vi "串口通信.vi"() -> ()   [LabVIEW 2014]
uses:
  <vilib>/Instr/_visa.llb/VISA Configure Serial Port (Instr).vi
  <vilib>/Utility/file.llb/Write To Spreadsheet File (string).vi
  <vilib>/sound2/lvsound2.llb/Sound File Read Open.vi
  <vilib>/sound2/lvsound2.llb/Sound File Read (DBL).vi
panel:
  in  "写入缓冲区":string="！0000?"
  in  "选项卡控件":enum32{"曲线图", "记录表", "设置"}(tab)
  out "湿度曲线 1":dbl(graph)
  out "温度曲线 1":dbl(graph)
  out "湿度曲线 2":dbl(graph)
  out "温度曲线 3":dbl(graph)
  out "湿度曲线 3":dbl(graph)
  out "温度曲线 2":dbl(graph)
  out "警报":bool
  out "湿度计 3":dbl(knob) scale=0.0..100.0
  out "警报":bool
  out "表格":string[][](table)
  out "湿度计  1":dbl(knob) scale=0.0..100.0
  out "湿度计 2":dbl(knob) scale=0.0..100.0
  out "温度计 1":dbl(slide) scale=0.0..100.0
  out "温度计 2":dbl(slide) scale=0.0..100.0
  out "温度计 3":dbl(slide) scale=0.0..100.0
  in  "创建表格":bool
  in  "选项卡控件 2":enum32{"开关选项", "上下限设置", "设置", "开发人员选项"}(tab)
  in  "自动模式":bool=TRUE
  in  "加热棒":bool
  in  "制冷片":bool
  in  "风扇":bool
  in  "报警灯":bool
  in  "湿度下限":u8(slide) scale=0.0..100.0
  in  "温度上限":u8(slide)=100 scale=0.0..100.0
  in  "温度下限":u8(slide) scale=0.0..100.0
  in  "湿度上限":u8(slide)=100 scale=0.0..100.0
  in  "Recipients 2":string="971661949@qq.com" caption="报警邮箱"
  in  "打开串口":bool
  in  "file path (dialog if empty)":path=path "d:/data.xls" caption="报表路径"
  in  "VISA resource name":refnum<visa-resource-name> caption="选择串口"
  in  "停止":bool
  out "火焰状态":string
  out "数据 4":string
  out "烟雾状态":string
  out "连接的字符串":string
  out "外人检测":string
  out "进入检测":string
  out "警报":bool
  in  "温湿度报警":bool
  in  "提示开关":bool=TRUE
  out "当前时间":timestamp format="%<%H:%M\n%Y年%m月%d>T日"
  out "数据 3":string
  out "输出数组":string[][](array[string])
  out "温度数据3":string
  out "湿度数据3":string
  out "数值 2":u8
  out "数据传输":i32
  out "湿度数据2":string
  out "温度数据2":string
  out "数据 2":string
  out "湿度数据1":string
  out "温度数据1":string
  out "数据 1":string
  in  "baud rate (9600)":u32=9600 caption="波特率(9600)"
  in  "parity (0:none)":enum16{"None", "Odd", "Even", "Mark", "Space"}(ring) caption="奇偶（0:无）"
  in  "data bits (8)":u16=8 caption="数据比特(8)" min=5 max=8 step=1
  in  "stop bits (10: 1 bit)":u16(ring)=10 caption="停止位（10: 1位）" items=["1.0"=10, "1.5"=15, "2.0"=20]
  in  "flow control (0:none)":u16(ring) caption="流控制（0:无）" items=["无", "XON/XOFF", "RTS/CTS", "XON/XOFF & RTS/CTS", "DTR/DSR", "XON/XOFF & DTR/DSR"]
  # "库房监控"
  # "使用图表实时反馈\n温湿度状况"
  # "这里有很全面的数据\n还可以将数据以表格形式保存到电脑"
  # "请在设置中选择串口位置"
  # "不要忘记核对信息哦"
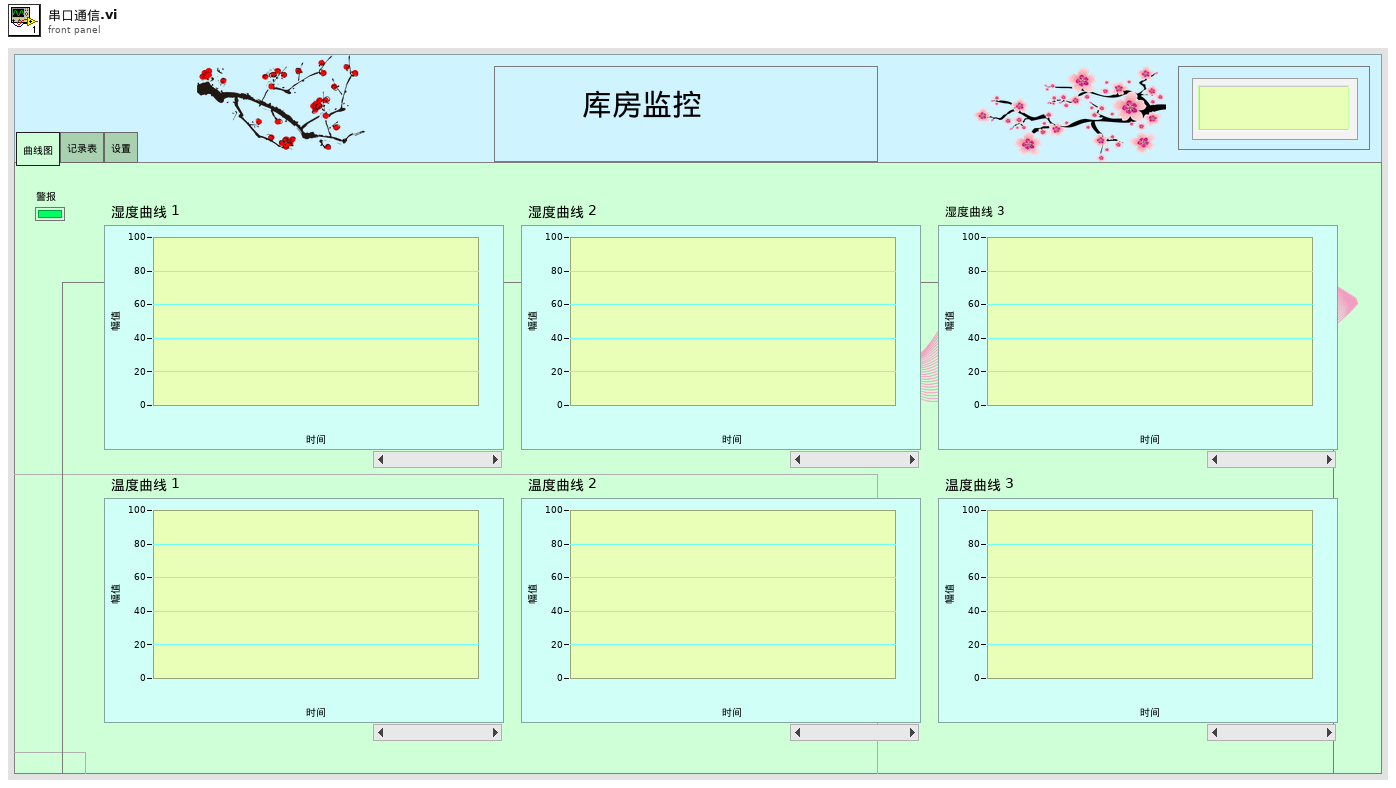
[diagram p1: front panel]
types:
  T1 = typedef "Sound File Refnum.ctl" = refnum<file>
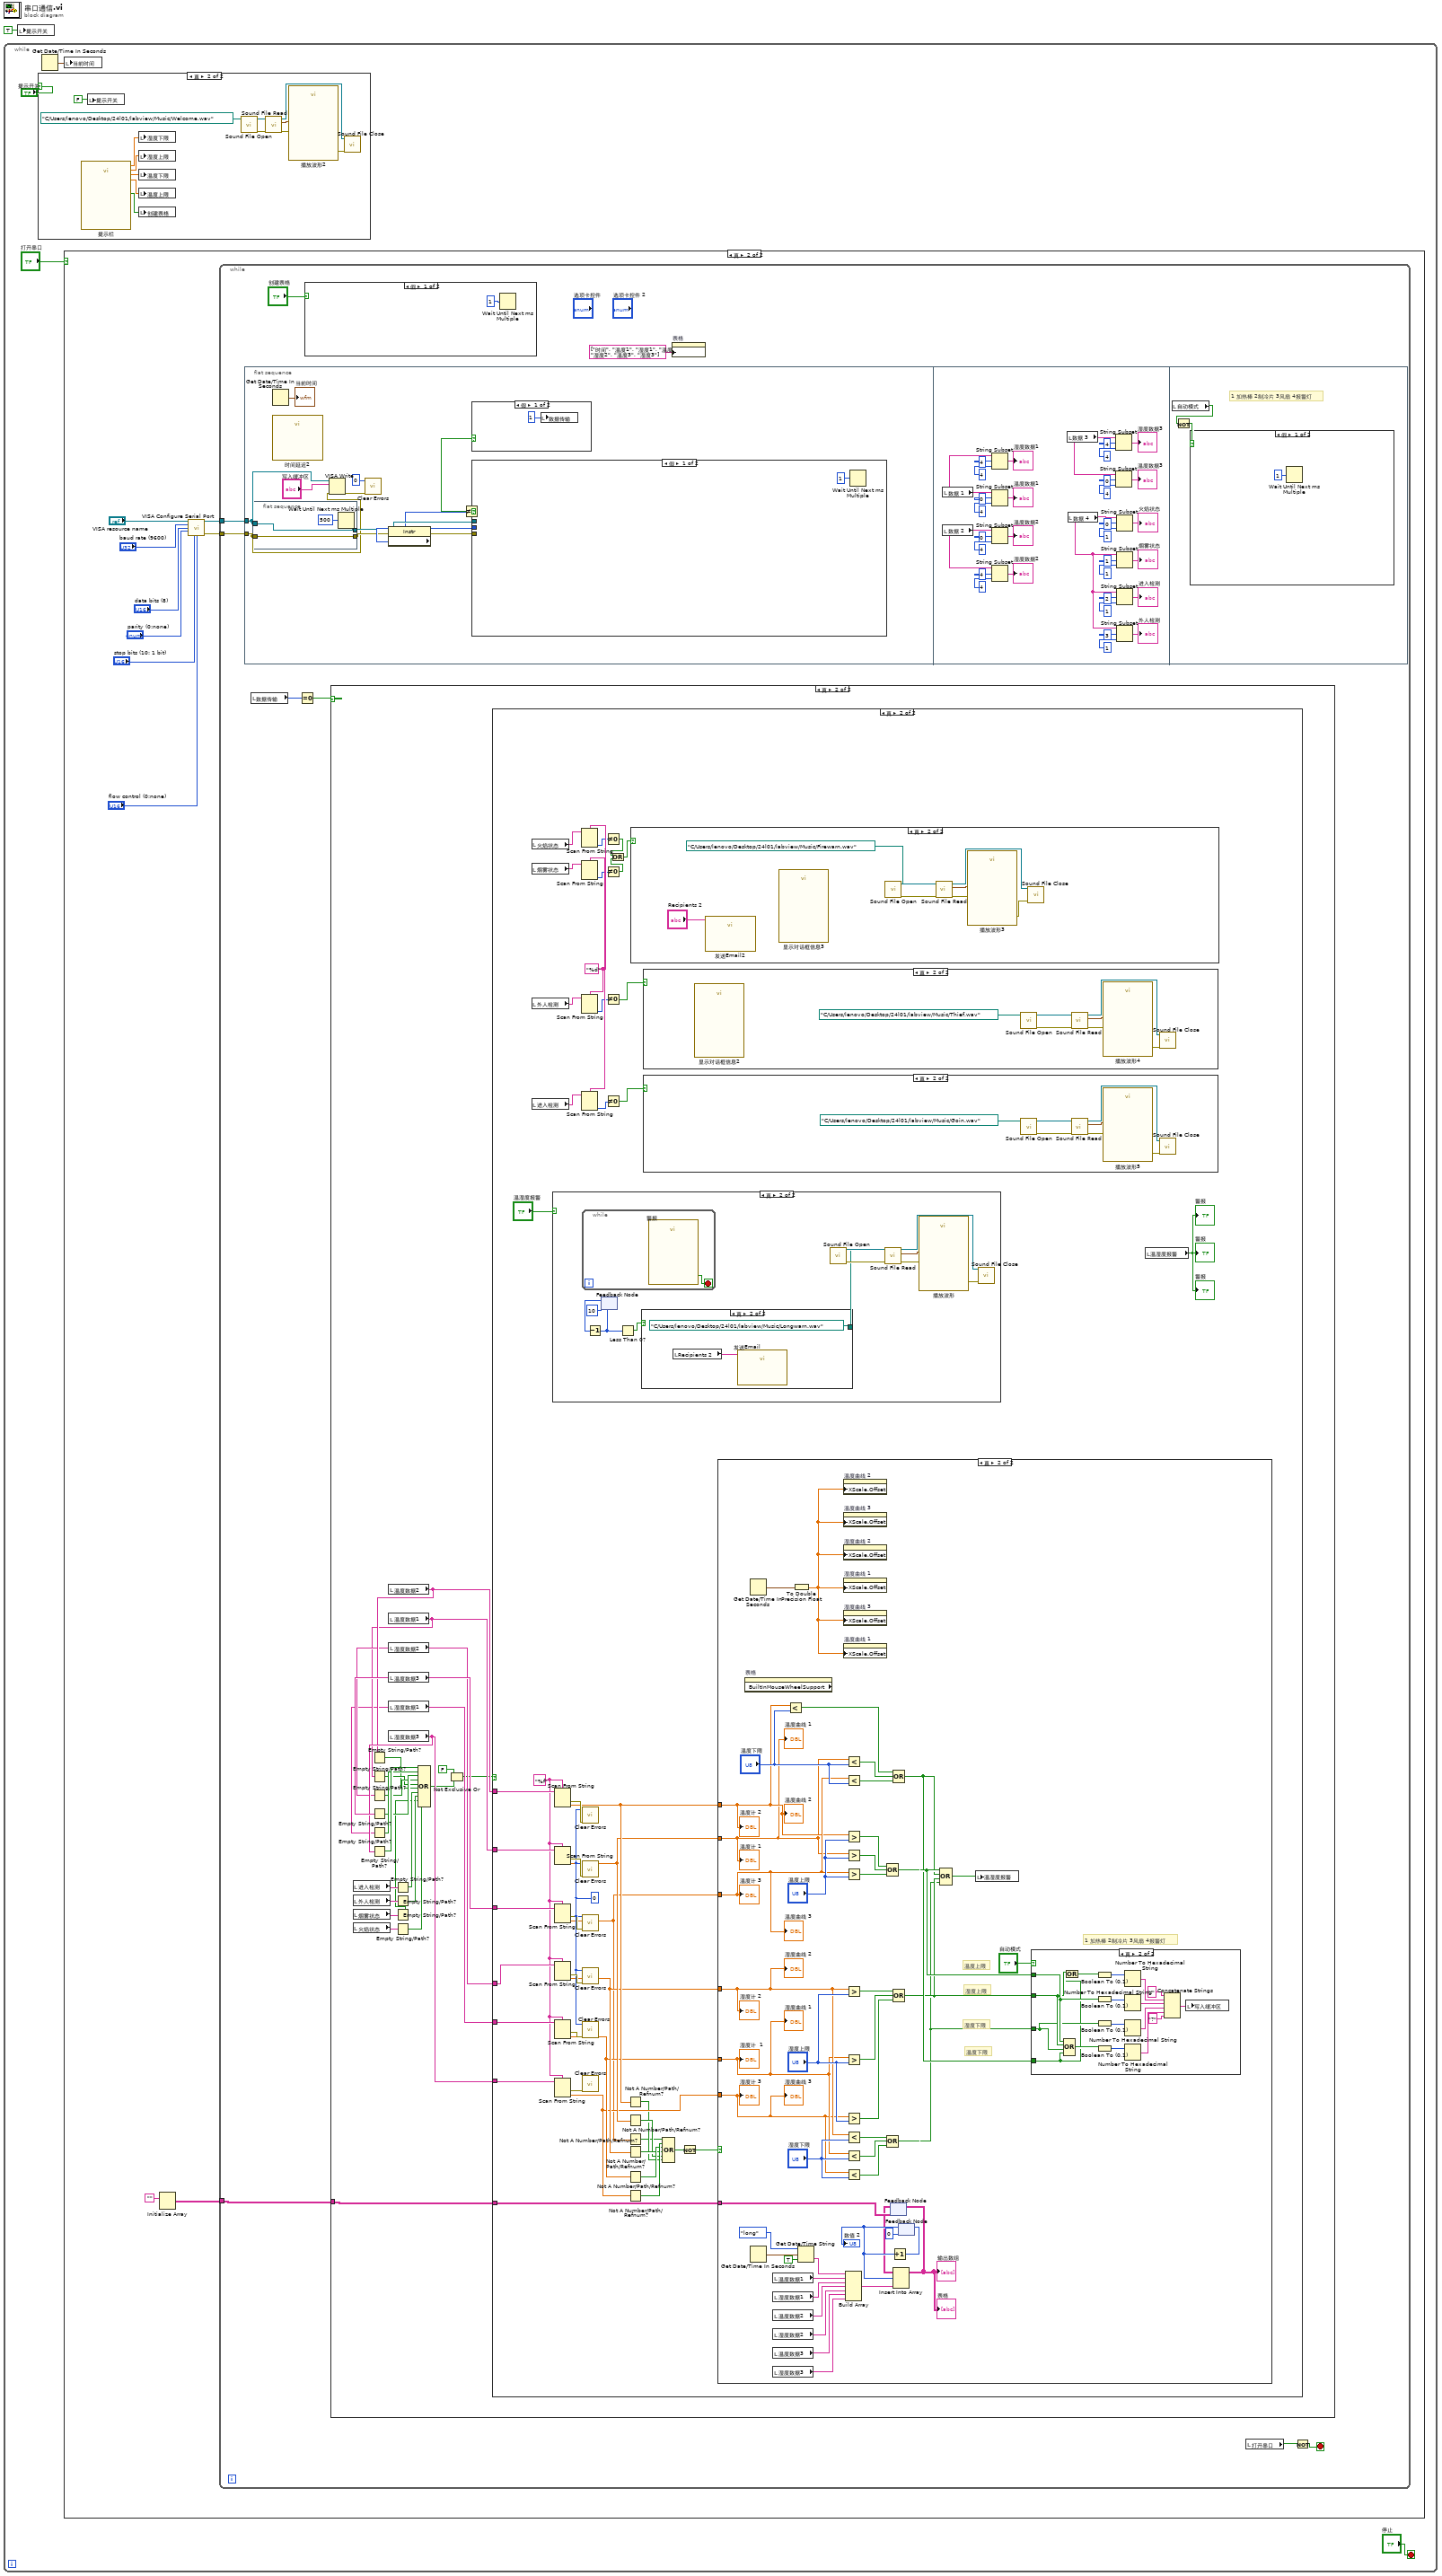
[diagram p0: block diagram]
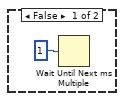
[diagram p3: hidden frame]
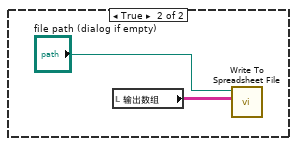
[diagram p4: hidden frame]
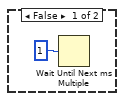
[diagram p5: hidden frame]
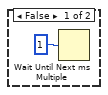
[diagram p11: hidden frame]
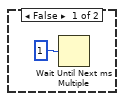
[diagram p12: hidden frame]
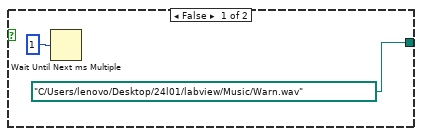
[diagram p13: hidden frame]
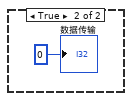
[diagram p14: hidden frame]
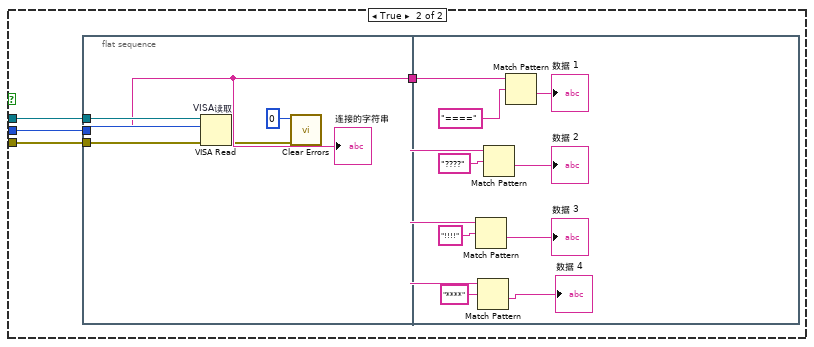
[diagram p15: hidden frame]
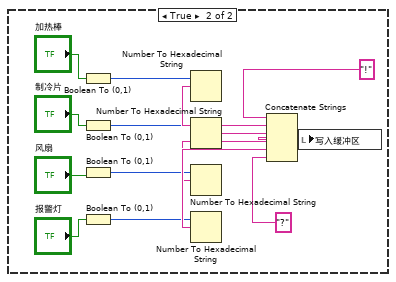
[diagram p16: hidden frame]
diagram:
  n1 = while {
    stop <- "停止" stop-if-true
    n2 = case shown="真" "提示开关" {
      frame False {
      }
      frame True {
        n3 = call "提示栏.vi"() -> ("是否创建报表"=w13:bool, "湿度下限"=w17:dbl, "湿度上限"=w16:dbl, "温度下限"=w15:dbl, "温度上限"=w14:dbl)  [unwired: 13 in, 2 out]
        n4 = local write "提示开关"(FALSE ("提示开关")) -> ()
        n5 = local write "湿度下限"(w17) -> ()
        n6 = local write "湿度上限"(w16) -> ()
        n7 = local write "温度下限"(w15) -> ()
        n8 = local write "温度上限"(w14) -> ()
        n9 = local write "创建表格"(w13) -> ()
        n10 = call-poly <vilib>:"Sound File Open.vi"("path"=path "C:/Users/lenovo/Desktop/24l01/labview/Music/Welcome.wav") -> ("error out"=w11:errorcluster, "sound file refnum"=w10:T1)  [unwired: 9 in]
        n11 = call-poly <vilib>:"Sound File Read.vi"("error in (no error)"=w11, "sound file refnum"=w10) -> ("error out"=w12:errorcluster, "data"=w9:waveform(dbl)[], "sound file refnum out"=w7:T1)  [unwired: 5 in, 2 out]
        n12 = call "播放波形2"("Data"=w9, "error in"=w12) -> ("error out"=w8:errorcluster)  [unwired: 17 in]
        n13 = call <vilib>:"Sound File Close.vi"("error in (no error)"=w8, "sound file refnum"=w7) -> ()  [unwired: 9 in, 1 out]
      }
    }
    n14 = Get Date/Time In Seconds() -> (seconds since 1Jan1904=w3:timestamp)
    n15 = local write "当前时间"(w3) -> ()
    n16 = case shown="真" "打开串口" {
      frame False {
        n17 = Wait Until Next ms Multiple(millisecond multiple=u32 1 ("毫秒倍数")) -> ()  [unwired: 1 out]
      }
      frame True {
        n18 = Initialize Array("") -> (w20:string[][])  [unwired: 2 in]
        n19 = call-poly "VISA Configure Serial Port"("VISA resource name"="VISA resource name", "baud rate (9600)"="baud rate (9600)", "data bits (8)"="data bits (8)", "parity (0:none)"="parity (0:none)", "stop bits (10: 1 bit)"="stop bits (10: 1 bit)", "flow control (0:none)"="flow control (0:none)") -> ("VISA resource name out"=w28:refnum<visa-resource-name>, "error out"=w29:errorcluster)  [unwired: 8 in]
        n20 = while {
          tunnel: w29 -> [w35]
          tunnel: w28 -> [w36]
          tunnel: w20 -> [w31]
          stop <- w37 stop-if-true
          n21 = flat-sequence {
            tunnel: w36 -> [w220]
            tunnel: w35 -> [w221]
            frame #0 {
              n22 = flat-sequence {
                tunnel: w220 -> [w232]
                tunnel: [w232] -> w224
                tunnel: [w230] -> w222
                tunnel: w221 -> [w230]
                frame #0 {
                  n23 = Wait Until Next ms Multiple(millisecond multiple=u32 500 ("毫秒倍数")) -> ()  [unwired: 1 out]
                }
              }
              n24 = Get Date/Time In Seconds() -> (seconds since 1Jan1904=→"当前时间":timestamp)
              n25 = call "时间延迟2"() -> ()  [unwired: 11 in, 1 out]
              n26 = VISA Write(VISA resource name=w220, write buffer="写入缓冲区", error in (no error)=w221) -> (error out=w218:errorcluster)  [unwired: 2 out]
              n27 = call <vilib>:"Clear Errors.vi"("error in (no error)"=w218, "specific error code to clear (0: all)"=0) -> ()  [unwired: 4 in, 2 out]
              n28 = property class="Instr"(reference=w224, error in=w222) -> (reference out=w226:refnum<visa-resource-name>, error out=w227:errorcluster, "Serial Settings:Number of Bytes at Serial Port"=w225:u32)
              n29 = Not Equal To 0?(x=w225) -> (x != 0?=w223:bool)
              n30 = case shown="假" w223 {
                frame False {
                  n31 = local write "数据传输"(1 ("数值")) -> ()
                }
                frame True {
                  "数据传输" <- 0 ("数值")
                }
              }
              n32 = case shown="假" w223 {
                tunnel: w227 -> [_ w236]
                tunnel: w226 -> [_ w237]
                tunnel: w225 -> [_ w235]
                frame False {
                  n33 = Wait Until Next ms Multiple(millisecond multiple=u32 1 ("毫秒倍数")) -> ()  [unwired: 1 out]
                }
                frame True {
                  n34 = flat-sequence {
                    tunnel: w236 -> [w242]
                    tunnel: w237 -> [w243]
                    tunnel: w235 -> [w241]
                    tunnel: [w240] -> w234
                    tunnel: w234 -> [w246]
                    frame #0 {
                      n35 = VISA Read "VISA读取"(VISA resource name=w243, byte count=w241, error in (no error)=w242) -> (read buffer=w240:string, error out=w239:errorcluster)  [unwired: 2 out]
                      "连接的字符串" <- w240
                      n36 = call <vilib>:"Clear Errors.vi"("error in (no error)"=w239, "specific error code to clear (0: all)"=0) -> ()  [unwired: 4 in, 2 out]
                    }
                    frame #1 {
                      n37 = Match Pattern(string=w246, regular expression="!!!!" ("正则表达式")) -> (after substring=→"数据 3":string)  [unwired: 1 in, 3 out]
                      n38 = Match Pattern(string=w246, regular expression="****" ("正则表达式")) -> (after substring=→"数据 4":string)  [unwired: 1 in, 3 out]
                      n39 = Match Pattern(string=w246, regular expression="????" ("正则表达式")) -> (after substring=→"数据 2":string)  [unwired: 1 in, 3 out]
                      n40 = Match Pattern(string=w246, regular expression="====" ("正则表达式")) -> (after substring=→"数据 1":string)  [unwired: 1 in, 3 out]
                    }
                  }
                }
              }
            }
            frame #1 {
              n41 = local read "数据 1"() -> (w282:string)
              n42 = local read "数据 2"() -> (w276:string)
              n43 = String Subset(string=w282, offset (0)=4 ("偏移量(0)"), length (rest)=4 ("长度（剩余）")) -> (substring=→"湿度数据1":string)
              n44 = String Subset(string=w282, offset (0)=0 ("偏移量(0)"), length (rest)=4 ("长度（剩余）")) -> (substring=→"温度数据1":string)
              n45 = String Subset(string=w276, offset (0)=0 ("偏移量(0)"), length (rest)=4 ("长度（剩余）")) -> (substring=→"温度数据2":string)
              n46 = String Subset(string=w276, offset (0)=4 ("长度（剩余）"), length (rest)=4 ("长度（剩余）")) -> (substring=→"湿度数据2":string)
              n47 = local read "数据 3"() -> (w268:string)
              n48 = local read "数据 4"() -> (w257:string)
              n49 = String Subset(string=w268, offset (0)=4 ("长度（剩余）"), length (rest)=4 ("长度（剩余）")) -> (substring=→"湿度数据3":string)
              n50 = String Subset(string=w268, offset (0)=0 ("长度（剩余）"), length (rest)=4 ("长度（剩余）")) -> (substring=→"温度数据3":string)
              n51 = String Subset(string=w257, offset (0)=0 ("偏移量(0)"), length (rest)=1 ("长度（剩余）")) -> (substring=→"火焰状态":string)
              n52 = String Subset(string=w257, offset (0)=1 ("偏移量(0)"), length (rest)=1 ("长度（剩余）")) -> (substring=→"烟雾状态":string)
              n53 = String Subset(string=w257, offset (0)=2 ("偏移量(0)"), length (rest)=1 ("长度（剩余）")) -> (substring=→"进入检测":string)
              n54 = String Subset(string=w257, offset (0)=3 ("偏移量(0)"), length (rest)=1 ("长度（剩余）")) -> (substring=→"外人检测":string)
            }
            frame #2 {
              # "1 加热棒 2制冷片 3风扇 4报警灯"
              n55 = local read "自动模式"() -> (w288:bool)
              n56 = Not(x=w288) -> (.not. x?=w287:bool)
              n57 = case shown="假" w287 {
                frame False {
                  n58 = Wait Until Next ms Multiple(millisecond multiple=u32 1 ("毫秒倍数")) -> ()  [unwired: 1 out]
                }
                frame True {
                  n59 = Boolean To (0,1)(Boolean="加热棒") -> (0, 1=w290:i16)
                  n60 = Boolean To (0,1)(Boolean="制冷片") -> (0, 1=w291:i16)
                  n61 = Boolean To (0,1)(Boolean="风扇") -> (0, 1=w292:i16)
                  n62 = Boolean To (0,1)(Boolean="报警灯") -> (0, 1=w293:i16)
                  n63 = Number To Hexadecimal String(2:w290) -> (0:w294:string)  [unwired: 1 in]
                  n64 = Number To Hexadecimal String(2:w291) -> (0:w295:string)  [unwired: 1 in]
                  n65 = Number To Hexadecimal String(2:w292) -> (0:w296:string)  [unwired: 1 in]
                  n66 = Number To Hexadecimal String(2:w293) -> (0:w297:string)  [unwired: 1 in]
                  n67 = Concatenate Strings("!" ("字符串"), w294, w295, w296, w297, "?" ("字符串")) -> (w300:string)
                  n68 = local write "写入缓冲区"(w300) -> ()
                }
              }
            }
          }
          n69 = local read "数据传输"() -> (w33:i32)
          n70 = Equal To 0?(x=w33) -> (x = 0?=w32:bool)
          n71 = case shown="假" "创建表格" {
            frame False {
              n72 = Wait Until Next ms Multiple(millisecond multiple=u32 1 ("毫秒倍数")) -> ()  [unwired: 1 out]
            }
            frame True {
              n73 = local read "输出数组"() -> (w41:string[][])
              n74 = call-poly <vilib>:"Write To Spreadsheet File.vi"("2D data"=w41, "file path (dialog if empty)"="file path (dialog if empty)") -> ()  [unwired: 6 in, 1 out]
            }
          }
          n75 = case shown="真" w32 {
            tunnel: w31 -> [_ w60]
            frame False {
              n76 = Wait Until Next ms Multiple(millisecond multiple=u32 1 ("毫秒倍数")) -> ()  [unwired: 1 out]
            }
            frame True {
              n77 = local read "进入检测"() -> (w50:string)
              n78 = local read "外人检测"() -> (w49:string)
              n79 = local read "烟雾状态"() -> (w48:string)
              n80 = local read "火焰状态"() -> (w47:string)
              n81 = local read "温度数据2"() -> (w64:string)
              n82 = Empty String/Path?(string/path=w64) -> (empty?=w54:bool)
              n83 = local read "温度数据1"() -> (w62:string)
              n84 = Empty String/Path?(string/path=w62) -> (empty?=w55:bool)
              n85 = local read "湿度数据2"() -> (w63:string)
              n86 = Empty String/Path?(string/path=w63) -> (empty?=w56:bool)
              n87 = local read "温度数据3"() -> (w66:string)
              n88 = Empty String/Path?(string/path=w66) -> (empty?=w57:bool)
              n89 = local read "湿度数据1"() -> (w61:string)
              n90 = Empty String/Path?(string/path=w61) -> (empty?=w58:bool)
              n91 = local read "湿度数据3"() -> (w65:string)
              n92 = Empty String/Path?(string/path=w65) -> (empty?=w59:bool)
              n93 = Empty String/Path?(string/path=w50) -> (empty?=w46:bool)
              n94 = Empty String/Path?(string/path=w49) -> (empty?=w45:bool)
              n95 = Empty String/Path?(string/path=w48) -> (empty?=w44:bool)
              n96 = Empty String/Path?(string/path=w47) -> (empty?=w43:bool)
              n97 = Compound Arithmetic op=OR(w59, w58, w57, w56, w55, w54, w46, w45, w44, w43) -> (w52:bool)
              n98 = Not Exclusive Or(1:w52, 2:FALSE ("x")) -> (0:w51:bool)
              n99 = case shown="真" w51 {
                tunnel: w61 -> [_ w110]
                tunnel: w62 -> [_ w111]
                tunnel: w63 -> [_ w109]
                tunnel: w64 -> [_ w108]
                tunnel: w65 -> [_ w107]
                tunnel: w66 -> [_ w106]
                tunnel: w60 -> [_ w104]
                frame False {
                }
                frame True {
                  w76 = "%d" ("格式字符串")
                  w97 = 0 ("specific error code to clear (0: all)")
                  w105 = "%f" ("格式字符串")
                  n100 = local read "火焰状态"() -> (w80:string)
                  n101 = local read "烟雾状态"() -> (w79:string)
                  n102 = local read "外人检测"() -> (w78:string)
                  n103 = local read "进入检测"() -> (w77:string)
                  n104 = case shown="真" "温湿度报警" {
                    frame False {
                      n105 = Wait Until Next ms Multiple(millisecond multiple=u32 1 ("毫秒倍数")) -> ()  [unwired: 1 out]
                    }
                    frame True {
                      n106 = while {
                        stop <- w215 stop-if-true
                        n107 = call "警报.vi"() -> ("确定"=w215:bool)  [unwired: 10 in, 1 out]
                      }
                      n108 = feedback #1(10) -> (w203:i32)
                      n109 = Decrement(x=w203) -> (x-1=w201:i32)
                      n110 = feedback-in #1(w201) -> ()
                      n111 = Less Than 0?(x=w201) -> (x < 0?=w202:bool)
                      n112 = case shown="真" w202 {
                        tunnel: [path "C:/Users/lenovo/Desktop/24l01/labview/Music/Warn.wav" ("path") path "C:/Users/lenovo/Desktop/24l01/labview/Music/Longwarn.wav" ("path")] -> w200
                        frame False {
                          n113 = Wait Until Next ms Multiple(millisecond multiple=u32 1 ("毫秒倍数")) -> ()  [unwired: 1 out]
                        }
                        frame True {
                          n114 = local read "Recipients 2"() -> (w213:string)
                          n115 = call "发送Email"("Recipients"=w213) -> ()  [unwired: 10 in, 1 out]
                        }
                      }
                      n116 = call-poly <vilib>:"Sound File Open.vi"("path"=w200) -> ("error out"=w209:errorcluster, "sound file refnum"=w208:T1)  [unwired: 9 in]
                      n117 = call-poly <vilib>:"Sound File Read.vi"("error in (no error)"=w209, "sound file refnum"=w208) -> ("error out"=w210:errorcluster, "data"=w207:waveform(dbl)[], "sound file refnum out"=w206:T1)  [unwired: 5 in, 2 out]
                      n118 = call "播放波形"("Data"=w207, "error in"=w210) -> ("error out"=w205:errorcluster)  [unwired: 17 in]
                      n119 = call <vilib>:"Sound File Close.vi"("error in (no error)"=w205, "sound file refnum"=w206) -> ()  [unwired: 9 in, 1 out]
                    }
                  }
                  n120 = Scan From String(format string=w105, input string=w108) -> (error out=w102:errorcluster, output 1=w96:dbl)  [unwired: 3 in, 2 out]
                  n121 = Scan From String(format string=w105, input string=w111) -> (error out=w103:errorcluster, output 1=w95:dbl)  [unwired: 3 in, 2 out]
                  n122 = Scan From String(format string=w105, input string=w106) -> (error out=w101:errorcluster, output 1=w91:dbl)  [unwired: 3 in, 2 out]
                  n123 = Scan From String(format string=w105, input string=w109) -> (error out=w99:errorcluster, output 1=w94:dbl)  [unwired: 3 in, 2 out]
                  n124 = Scan From String(format string=w105, input string=w110) -> (error out=w98:errorcluster, output 1=w93:dbl)  [unwired: 3 in, 2 out]
                  n125 = Scan From String(format string=w105, input string=w107) -> (error out=w100:errorcluster, output 1=w92:dbl)  [unwired: 3 in, 2 out]
                  n126 = Scan From String(format string=w76, input string=w80) -> (output 1=w67:i32)  [unwired: 3 in, 3 out]
                  n127 = Scan From String(format string=w76, input string=w79) -> (output 1=w75:i32)  [unwired: 3 in, 3 out]
                  n128 = Scan From String(format string=w76, input string=w78) -> (output 1=w74:i32)  [unwired: 3 in, 3 out]
                  n129 = Scan From String(format string=w76, input string=w77) -> (output 1=w73:i32)  [unwired: 3 in, 3 out]
                  n130 = call <vilib>:"Clear Errors.vi"("error in (no error)"=w102, "specific error code to clear (0: all)"=w97) -> ()  [unwired: 4 in, 2 out]
                  n131 = call <vilib>:"Clear Errors.vi"("error in (no error)"=w103, "specific error code to clear (0: all)"=w97) -> ()  [unwired: 4 in, 2 out]
                  n132 = call <vilib>:"Clear Errors.vi"("error in (no error)"=w101, "specific error code to clear (0: all)"=w97) -> ()  [unwired: 4 in, 2 out]
                  n133 = call <vilib>:"Clear Errors.vi"("error in (no error)"=w99, "specific error code to clear (0: all)"=w97) -> ()  [unwired: 4 in, 2 out]
                  n134 = call <vilib>:"Clear Errors.vi"("error in (no error)"=w98, "specific error code to clear (0: all)"=w97) -> ()  [unwired: 4 in, 2 out]
                  n135 = call <vilib>:"Clear Errors.vi"("error in (no error)"=w100) -> ()  [unwired: 5 in, 2 out]
                  n136 = Not Equal To 0?(x=w67) -> (x != 0?=w69:bool)
                  n137 = Not Equal To 0?(x=w75) -> (x != 0?=w70:bool)
                  n138 = Not Equal To 0?(x=w74) -> (x != 0?=w72:bool)
                  n139 = Not Equal To 0?(x=w73) -> (x != 0?=w71:bool)
                  n140 = Or(x=w69, y=w70) -> (x .or. y?=w68:bool)
                  n141 = Not A Number/Path/Refnum?(number/path/refnum=w96) -> (NaN/Path/Refnum?=w86:bool)
                  n142 = Not A Number/Path/Refnum?(number/path/refnum=w95) -> (NaN/Path/Refnum?=w87:bool)
                  n143 = Not A Number/Path/Refnum?(number/path/refnum=w91) -> (NaN/Path/Refnum?=w85:bool)
                  n144 = Not A Number/Path/Refnum?(number/path/refnum=w94) -> (NaN/Path/Refnum?=w88:bool)
                  n145 = Not A Number/Path/Refnum?(number/path/refnum=w93) -> (NaN/Path/Refnum?=w89:bool)
                  n146 = Not A Number/Path/Refnum?(number/path/refnum=w92) -> (NaN/Path/Refnum?=w90:bool)
                  n147 = case shown="真" w68 {
                    frame False {
                    }
                    frame True {
                      n148 = call "发送Email2"("Recipients"="Recipients 2") -> ()  [unwired: 10 in, 1 out]
                      n149 = call "显示对话框信息3"() -> ()  [unwired: 10 in, 2 out]
                      n150 = call-poly <vilib>:"Sound File Open.vi"("path"=path "C:/Users/lenovo/Desktop/24l01/labview/Music/Firewarn.wav") -> ("error out"=w132:errorcluster, "sound file refnum"=w131:T1)  [unwired: 9 in]
                      n151 = call-poly <vilib>:"Sound File Read.vi"("error in (no error)"=w132, "sound file refnum"=w131) -> ("error out"=w133:errorcluster, "data"=w130:waveform(dbl)[], "sound file refnum out"=w129:T1)  [unwired: 5 in, 2 out]
                      n152 = call "播放波形3"("Data"=w130, "error in"=w133) -> ("error out"=w128:errorcluster)  [unwired: 17 in]
                      n153 = call <vilib>:"Sound File Close.vi"("error in (no error)"=w128, "sound file refnum"=w129) -> ()  [unwired: 9 in, 1 out]
                    }
                  }
                  n154 = case shown="真" w72 {
                    frame False {
                    }
                    frame True {
                      n155 = call "显示对话框信息2"() -> ()  [unwired: 10 in, 2 out]
                      n156 = call-poly <vilib>:"Sound File Open.vi"("path"=path "C:/Users/lenovo/Desktop/24l01/labview/Music/Thief.wav") -> ("error out"=w124:errorcluster, "sound file refnum"=w123:T1)  [unwired: 9 in]
                      n157 = call-poly <vilib>:"Sound File Read.vi"("error in (no error)"=w124, "sound file refnum"=w123) -> ("error out"=w125:errorcluster, "data"=w122:waveform(dbl)[], "sound file refnum out"=w121:T1)  [unwired: 5 in, 2 out]
                      n158 = call "播放波形4"("Data"=w122, "error in"=w125) -> ("error out"=w120:errorcluster)  [unwired: 17 in]
                      n159 = call <vilib>:"Sound File Close.vi"("error in (no error)"=w120, "sound file refnum"=w121) -> ()  [unwired: 9 in, 1 out]
                    }
                  }
                  n160 = case shown="真" w71 {
                    frame False {
                    }
                    frame True {
                      n161 = call-poly <vilib>:"Sound File Open.vi"("path"=path "C:/Users/lenovo/Desktop/24l01/labview/Music/Goin.wav") -> ("error out"=w117:errorcluster, "sound file refnum"=w116:T1)  [unwired: 9 in]
                      n162 = call-poly <vilib>:"Sound File Read.vi"("error in (no error)"=w117, "sound file refnum"=w116) -> ("error out"=w118:errorcluster, "data"=w115:waveform(dbl)[], "sound file refnum out"=w114:T1)  [unwired: 5 in, 2 out]
                      n163 = call "播放波形5"("Data"=w115, "error in"=w118) -> ("error out"=w113:errorcluster)  [unwired: 17 in]
                      n164 = call <vilib>:"Sound File Close.vi"("error in (no error)"=w113, "sound file refnum"=w114) -> ()  [unwired: 9 in, 1 out]
                    }
                  }
                  n165 = Compound Arithmetic op=OR(w85, w90, w89, w88, w87, w86) -> (w82:bool)
                  n166 = Not(x=w82) -> (.not. x?=w81:bool)
                  n167 = case shown="真" w81 {
                    tunnel: w104 -> [_ w180]
                    tunnel: w96 -> [_ w157]
                    tunnel: w95 -> [_ w156]
                    tunnel: w94 -> [_ w159]
                    tunnel: w93 -> [_ w154]
                    tunnel: w92 -> [_ w152]
                    tunnel: w91 -> [_ w158]
                    frame False {
                    }
                    frame True {
                      # "1 加热棒 2制冷片 3风扇 4报警灯"
                      # "湿度下限"
                      # "湿度上限"
                      # "温度下限"
                      # "温度上限"
                      n168 = property on="表格" class="Tbl (严格)" props=["BuiltInMouseWheelSupport"]() -> ()  [unwired: 2 in, 3 out]
                      n169 = Get Date/Time In Seconds() -> (seconds since 1Jan1904=w155:timestamp)
                      n170 = Get Date/Time In Seconds() -> (seconds since 1Jan1904=w177:timestamp)
                      n171 = local read "温度数据1"() -> (w165:string)
                      n172 = local read "湿度数据1"() -> (w176:string)
                      n173 = local read "温度数据2"() -> (w171:string)
                      n174 = local read "湿度数据2"() -> (w170:string)
                      n175 = local read "温度数据3"() -> (w169:string)
                      n176 = local read "湿度数据3"() -> (w168:string)
                      n177 = Less?(x=w157, y="温度下限") -> (x < y?=w148:bool)
                      n178 = To Double Precision Float(number=w155) -> (double precision float=w153:dbl)
                      n179 = Get Date/Time String(date format (0)=enum16{"short", "long", "abbreviated"}."long" ("日期格式(0)"), seconds (now)=w177, want seconds? (F)=TRUE ("需要秒？(F)")) -> (time string=w164:string)  [unwired: 1 out]
                      n180 = property on="温度曲线 2" class="WFChart (严格)"("XScale.Offset"=w153) -> ()  [unwired: 2 in, 2 out]
                      n181 = property on="温度曲线 3" class="WFChart (严格)"("XScale.Offset"=w153) -> ()  [unwired: 2 in, 2 out]
                      n182 = property on="湿度曲线 2" class="WFChart (严格)"("XScale.Offset"=w153) -> ()  [unwired: 2 in, 2 out]
                      n183 = property on="湿度曲线 1" class="WFChart (严格)"("XScale.Offset"=w153) -> ()  [unwired: 2 in, 2 out]
                      n184 = property on="湿度曲线 3" class="WFChart (严格)"("XScale.Offset"=w153) -> ()  [unwired: 2 in, 2 out]
                      n185 = property on="温度曲线 1" class="WFChart (严格)"("XScale.Offset"=w153) -> ()  [unwired: 2 in, 2 out]
                      n186 = Build Array(w164, w165, w176, w171, w170, w169, w168) -> (w166:string[])
                      n187 = Less?(x=w156, y="温度下限") -> (x < y?=w147:bool)
                      n188 = Less?(x=w158, y="温度下限") -> (x < y?=w146:bool)
                      n189 = Greater?(x=w157, y="温度上限") -> (0:w151:bool)
                      n190 = Greater?(x=w156, y="温度上限") -> (0:w150:bool)
                      n191 = Greater?(x=w158, y="温度上限") -> (0:w149:bool)
                      n192 = Greater?(x=w159, y="湿度上限") -> (0:w145:bool)
                      n193 = Greater?(x=w154, y="湿度上限") -> (0:w144:bool)
                      n194 = Greater?(x=w152, y="湿度上限") -> (0:w143:bool)
                      n195 = Less?(x=w159, y="湿度下限") -> (x < y?=w142:bool)
                      n196 = Less?(x=w154, y="湿度下限") -> (x < y?=w141:bool)
                      n197 = Less?(x=w152, y="湿度下限") -> (x < y?=w140:bool)
                      n198 = Compound Arithmetic op=OR(w151, w150, w149) -> (w138:bool)
                      n199 = Compound Arithmetic op=OR(w142, w141, w140) -> (w135:bool)
                      n200 = feedback #2(w180) -> (w172:string[][])
                      n201 = Compound Arithmetic op=OR(w148, w147, w146) -> (w137:bool)
                      n202 = Compound Arithmetic op=OR(w145, w144, w143) -> (w136:bool)
                      n203 = feedback #3(0) -> (w174:i32)
                      "数值 2" <- w174
                      n204 = Increment(x=w174) -> (x+1=w175:i32)
                      n205 = Insert Into Array(array=w172, index (row)=w174, new element=w166) -> (w167:string[][])  [unwired: 1 in]
                      "表格" <- w167
                      "输出数组" <- w167
                      n206 = feedback-in #2(w167) -> ()
                      n207 = feedback-in #3(w175) -> ()
                      n208 = Compound Arithmetic op=OR(w138, w137, w136, w135) -> (w139:bool)
                      n209 = local write "温湿度报警"(w139) -> ()
                      n210 = case shown="真" "自动模式" {
                        tunnel: w138 -> [_ w185]
                        tunnel: w137 -> [_ w182]
                        tunnel: w136 -> [_ w184]
                        tunnel: w135 -> [_ w183]
                        frame False {
                          n211 = Wait Until Next ms Multiple(millisecond multiple=u32 1 ("毫秒倍数")) -> ()  [unwired: 1 out]
                        }
                        frame True {
                          n212 = Compound Arithmetic op=OR(w185, w184, w183, w182) -> (w186:bool)
                          n213 = Or(x=w184, y=w182) -> (x .or. y?=w187:bool)
                          n214 = Boolean To (0,1)(Boolean=w187) -> (0, 1=w198:i16)
                          n215 = Boolean To (0,1)(Boolean=w185) -> (0, 1=w197:i16)
                          n216 = Boolean To (0,1)(Boolean=w183) -> (0, 1=w196:i16)
                          n217 = Boolean To (0,1)(Boolean=w186) -> (0, 1=w195:i16)
                          n218 = Number To Hexadecimal String(2:w198) -> (0:w194:string)  [unwired: 1 in]
                          n219 = Number To Hexadecimal String(2:w197) -> (0:w193:string)  [unwired: 1 in]
                          n220 = Number To Hexadecimal String(2:w196) -> (0:w192:string)  [unwired: 1 in]
                          n221 = Number To Hexadecimal String(2:w195) -> (0:w191:string)  [unwired: 1 in]
                          n222 = Concatenate Strings("!" ("字符串"), w194, w193, w192, w191, "?" ("字符串")) -> (w190:string)
                          n223 = local write "写入缓冲区"(w190) -> ()
                        }
                      }
                      "温度计 1" <- w156
                      "湿度计  1" <- w154
                      "温度曲线 2" <- w157
                      "湿度曲线 3" <- w152
                      "温度曲线 3" <- w158
                      "湿度计 2" <- w159
                      "温度计 2" <- w157
                      "温度计 3" <- w158
                      "湿度曲线 2" <- w159
                      "温度曲线 1" <- w156
                      "湿度曲线 1" <- w154
                      "湿度计 3" <- w152
                    }
                  }
                  n224 = local read "温湿度报警"() -> (→"警报" →"警报" →"警报":bool)
                }
              }
            }
          }
          n225 = property on="表格" class="Tbl (严格)"("Column Headers[]"=string[] ["时间", "温度1", "湿度1", "温度2", "湿度2", "温度3", "湿度3"] ("列首字符串[]")) -> ()  [unwired: 2 in, 2 out]
          n226 = local read "打开串口"() -> (w38:bool)
          n227 = Not(x=w38) -> (.not. x?=w37:bool)
        }
      }
    }
  }
  n228 = local write "提示开关"(TRUE ("布尔")) -> ()
